vi "Is Counter Task.vi"(8 "error in":errorcluster, 11 "Task":refnum<k21>) -> (0 "error out":errorcluster, 2 "Is Counter Task":bool, 3 "Task":refnum<k21>)   [LabVIEW 2022 SP3]
doc: "Given a task, this VI will determine if the channels in the task are Counter Input or Counter Output channels."
uses:
  <resource>/objmgr/daqmx.rc
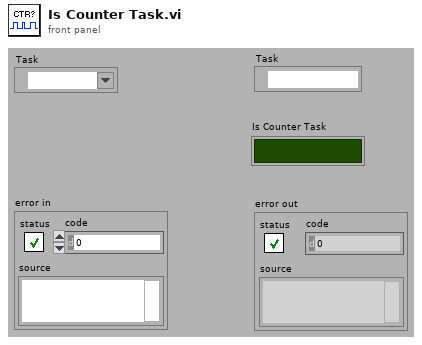
[diagram p1: front panel]
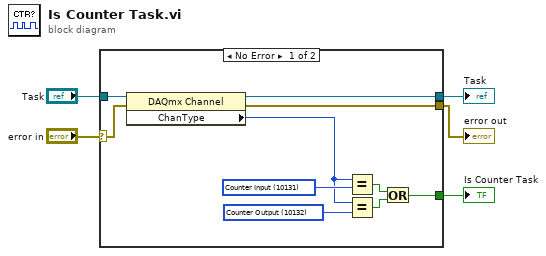
[diagram p0: block diagram]
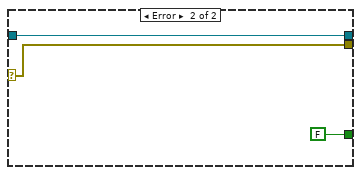
[diagram p2: hidden frame]
diagram:
  n1 = case shown="No Error" "error in" {
    selector: "error in" -> [w6 w17]
    tunnel: "Task" -> [w15 w18]
    tunnel: [w14 w18] -> w4
    tunnel: [w13 w17] -> w3
    tunnel: [w8 FALSE] -> w2
    frame No Error {
      w11 = 10132 items=["Analog Input"=10100, "Analog Output"=10102, "Digital Input"=10151, "Digital Output"=10153, "Counter Input"=10131, "Counter Output"=10132] ("ChanType")
      w12 = 10131 items=["Analog Input"=10100, "Analog Output"=10102, "Digital Input"=10151, "Digital Output"=10153, "Counter Input"=10131, "Counter Output"=10132] ("ChanType")
      n2 = property class="DAQmx Channel"(reference=w15, error in=w6) -> (reference out=w14:refnum<k21>, error out=w13:errorcluster, "ChanType"=w7:i32)
      n3 = Equal?(x=w7, y=w12) -> (x = y?=w10:bool)
      n4 = Equal?(x=w7, y=w11) -> (x = y?=w9:bool)
      n5 = Or(x=w10, y=w9) -> (x .or. y?=w8:bool)
    }
    frame Error {
    }
  }
  "error out" <- w3
  "Task" <- w4
  "Is Counter Task" <- w2
